vi "replaceInElementValue.vi"(7 "replaceElementIn":string, 8 "error in (no error)":errorcluster, 9 "replaceWithValue":string, 10 "replacementElementName":string, 11 "xmlNode in":refnum<class "xmlNode.lvclass">) -> (0 "error out":errorcluster, 2 "replacementxXmlNode":refnum<class "xmlNode.lvclass">, 3 "xmlNode out":refnum<class "xmlNode.lvclass">)   [LabVIEW 2011, in "Tools.lvlib" / "xml.lvlib" / "xmlNode.lvclass"]
uses:
  xmlNode.lvclass
  XmlParser.lvclass
panel:
  out "found?":bool=TRUE
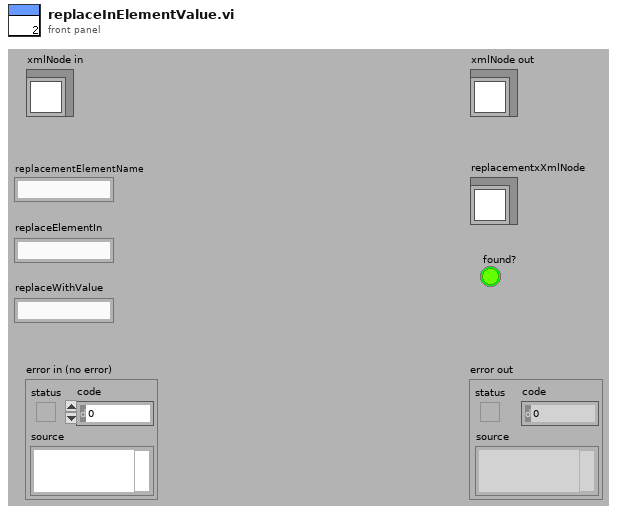
[diagram p1: front panel]
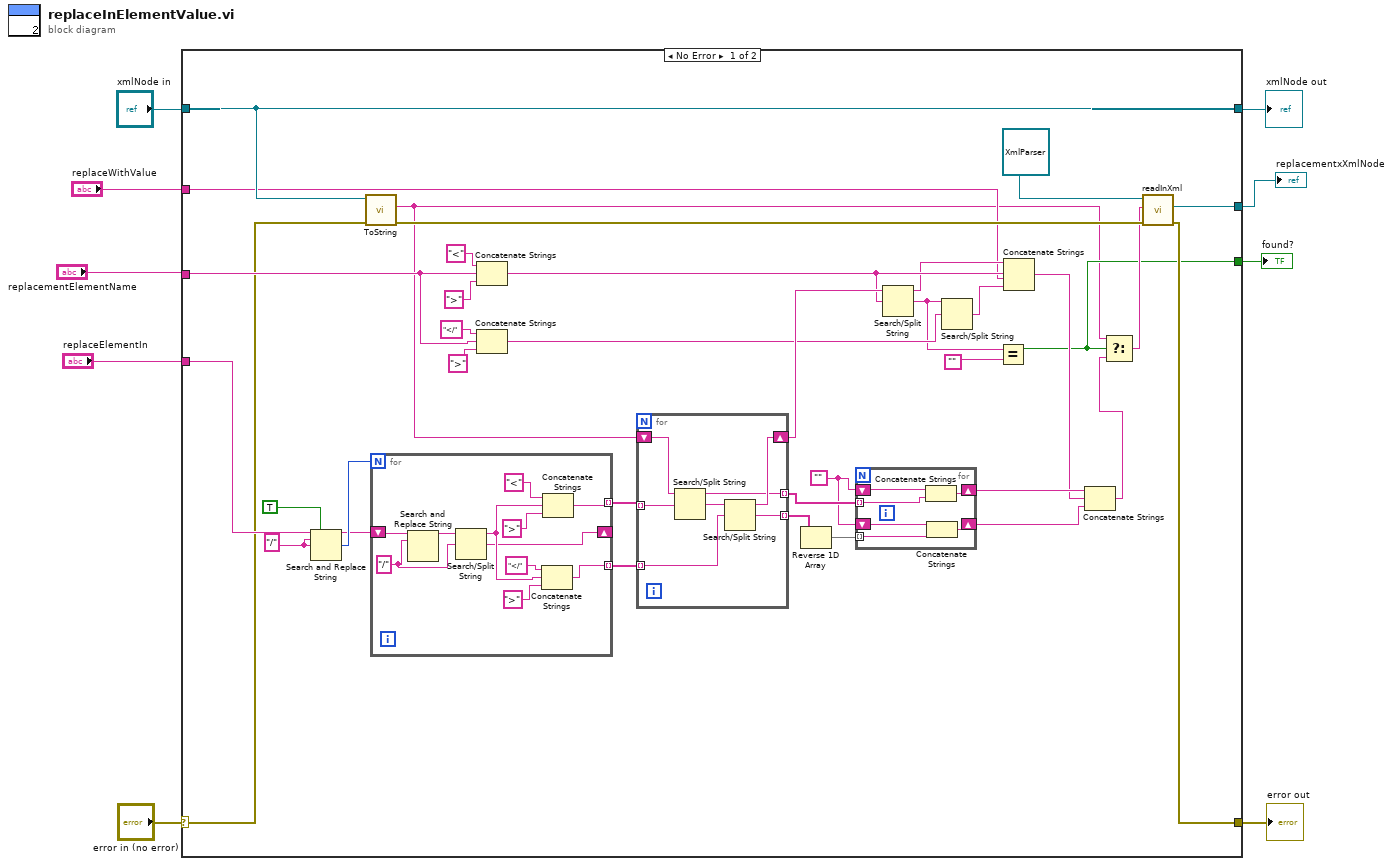
[diagram p0: block diagram]
diagram:
  n1 = case shown="No Error" "error in (no error)" {
    selector: "error in (no error)" -> [w35 w72]
    tunnel: [w19 w72] -> w8
    tunnel: [w36 w71] -> w6
    tunnel: "xmlNode in" -> [w36 w71]
    tunnel: "replaceElementIn" -> [w38 _]
    tunnel: "replacementElementName" -> [w37 _]
    tunnel: "replaceWithValue" -> [w14 _]
    tunnel: [w18 _] -> w2
    tunnel: [w11 _] -> w1
    frame No Error {
      w26 = ""
      w33 = "/"
      n2 = Search and Replace String(replace all?=TRUE, input string=w38, search string=w33, replace string=w33) -> (result string=w41:string, number of replacements=w42:i32)  [unwired: 4 in, 2 out]
      n3 = call-dynamic "ToString.vi"("error in (no error)"=w35, "xmlNode in"=w36) -> ("error out"=w20:errorcluster, "xml"=w10:string)  [unwired: 7 in, 1 out]
      n4 = for {
        N: w42 -> [_]
        tunnel: [w55] -> w40 mode=indexing
        tunnel: [w54] -> w39 mode=indexing
        shift-right: [w53] -> _
        shift-left: w41 -> [w56]
        w63 = "/"
        n5 = Search and Replace String(input string=w56, search string=w63) -> (result string=w62:string)  [unwired: 6 in, 3 out]
        n6 = Search/Split String(string=w62, search string/char (-)=w63) -> (substring before match=w57:string, match + rest of string=w53:string)  [unwired: 1 in, 1 out]
        n7 = Concatenate Strings("</", w57, ">") -> (w54:string)
        n8 = Concatenate Strings("<", w57, ">") -> (w55:string)
      }
      n9 = Concatenate Strings("<", w37, ">") -> (w30:string)
      n10 = Concatenate Strings("</", w37, ">") -> (w31:string)
      n11 = for {
        tunnel: w40 -> [w69] mode=indexing
        tunnel: w39 -> [w67] mode=indexing
        shift-right: [w66] -> w32
        shift-left: w10 -> [w70]
        tunnel: [w65] -> w28 mode=indexing
        tunnel: [w64] -> w27 mode=indexing
        n12 = Search/Split String(string=w70, search string/char (-)=w69) -> (substring before match=w65:string, match + rest of string=w68:string)  [unwired: 1 in, 1 out]
        n13 = Search/Split String(string=w68, search string/char (-)=w67) -> (substring before match=w66:string, match + rest of string=w64:string)  [unwired: 1 in, 1 out]
      }
      n14 = Reverse 1D Array(array=w27) -> (reversed array=w25:string[])
      n15 = for {
        tunnel: w28 -> [w51] mode=indexing
        tunnel: w25 -> [w49] mode=indexing
        shift-right: [w50] -> w24
        shift-left: w26 -> [w52]
        shift-right: [w47] -> w22
        shift-left: w26 -> [w48]
        n16 = Concatenate Strings(w52, w51) -> (w50:string)
        n17 = Concatenate Strings(w48, w49) -> (w47:string)
      }
      n18 = Search/Split String(string=w32, search string/char (-)=w30) -> (substring before match=w17:string, match + rest of string=w16:string)  [unwired: 1 in, 1 out]
      n19 = Search/Split String(string=w16, search string/char (-)=w31) -> (match + rest of string=w29:string)  [unwired: 1 in, 2 out]
      n20 = Equal?(x=w16, y="") -> (x = y?=w11:bool)
      n21 = Concatenate Strings(w17, w30, w14, w29) -> (w23:string)
      n22 = Concatenate Strings(w24, w23, w22) -> (w12:string)
      n23 = Select(t=w10, s=w11, f=w12) -> (s? t:f=w13:string)
      n24 = call "readInXml.vi"("error in (no error)"=w20, "xmlString"=w13, "XmlParser in"=refnum<class "XmlParser.lvclass"> refnum ("Tools.lvlib:XmlParser.lvclass")) -> ("error out"=w19:errorcluster, "xmlNode"=w18:refnum<class "xmlNode.lvclass">)  [unwired: 6 in, 1 out]
    }
    frame Error {
    }
  }
  "error out" <- w8
  "xmlNode out" <- w6
  "replacementxXmlNode" <- w2
  "found?" <- w1
